vi "Set caseStructure Position and Size.vi"() -> ()   [LabVIEW 2012]
uses:
  <vilib>/Utility/miscctls.llb/LVBoundsTypeDef.ctl
panel:
  in  "Project Path":path
  in  "My Computer?":bool
  in  "Path":path
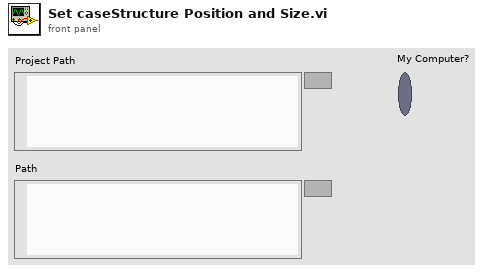
[diagram p1: front panel]
types:
  T1 = typedef "LVBoundsTypeDef.ctl" = cluster{"Width":u32, "Height":u32}
  T2 = typedef "LVPositionTypeDef.ctl" = cluster{"Left":i32, "Top":i32}
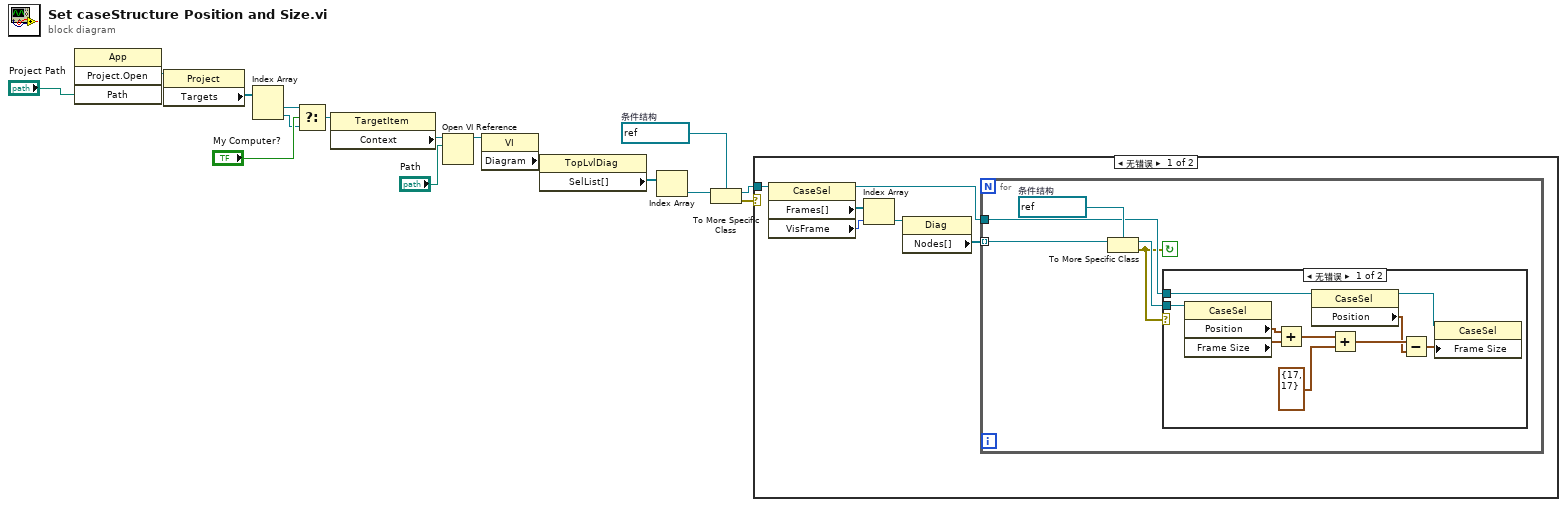
[diagram p0: block diagram]
diagram:
  w3 = refnum<vi> refnum  # 条件结构
  n1 = invoke class="App" method="Project.Open"("Path"="Project Path") -> ("Project:Open"=w15:refnum<vi>)  [unwired: 3 in, 3 out]
  n2 = property class="Project"(reference=w15) -> ("Targets"=w14:refnum<vi>[])  [unwired: 1 in, 2 out]
  n3 = Index Array(array=w14) -> (element #1=w11:refnum<vi>, element #2=w10:refnum<vi>)  [unwired: 2 in]
  n4 = Select(t=w11, s="My Computer?", f=w10) -> (s? t:f=w9:refnum<vi>)
  n5 = property class="TargetItem"(reference=w9) -> ("Context"=w8:refnum<vi>)  [unwired: 1 in, 2 out]
  n6 = Open VI Reference(application reference (local)=w8, vi path="Path") -> (vi reference=w7:refnum<vi>)  [unwired: 4 in, 1 out]
  n7 = property class="VI"(reference=w7) -> ("Diagram"=w6:refnum<vi>)  [unwired: 1 in, 2 out]
  n8 = property class="TopLvlDiag"(reference=w6) -> ("SelList[]"=w5:refnum<vi>[])  [unwired: 1 in, 2 out]
  n9 = Index Array(array=w5) -> (element=w4:refnum<vi>)  [unwired: 1 in]
  n10 = To More Specific Class(target class=w3, reference=w4) -> (specific class reference=w1:refnum<vi>, error out=w2:errorcluster)  [unwired: 1 in]
  n11 = case shown="无错误" w2 {
    tunnel: w1 -> [w22 _]
    frame No Error {
      n12 = property class="CaseSel"(reference=w22) -> (reference out=w19:refnum<vi>, "Frames[]"=w21:refnum<vi>[], "VisFrame"=w20:u32)  [unwired: 1 in, 1 out]
      n13 = Index Array(array=w21, index=w20) -> (element=w18:refnum<vi>)
      n14 = property class="Diag"(reference=w18) -> ("Nodes[]"=w17:refnum<vi>[])  [unwired: 1 in, 2 out]
      n15 = for {
        tunnel: w19 -> [w25]
        tunnel: w17 -> [w24] mode=indexing
        stop <- w23 continue-if-true
        w27 = refnum<vi> refnum  # 条件结构
        n16 = To More Specific Class(target class=w27, reference=w24) -> (specific class reference=w26:refnum<vi>, error out=w23:errorcluster)  [unwired: 1 in]
        n17 = case shown="无错误" w23 {
          tunnel: w26 -> [w37 _]
          tunnel: w25 -> [w31 _]
          frame No Error {
            n18 = property class="CaseSel"(reference=w37) -> ("Position"=w36:T2, "Frame Size"=w35:T1)  [unwired: 1 in, 2 out]
            n19 = Add(x=w36, y=w35) -> (x+y=w34:T1)
            n20 = property class="CaseSel"(reference=w31) -> (reference out=w30:refnum<vi>, "Position"=w28:T2)  [unwired: 1 in, 1 out]
            n21 = Add(x=w34, y=T1 {"Width"=17, "Height"=17}) -> (x+y=w32:T1)
            n22 = Subtract(x=w32, y=w28) -> (x-y=w29:T1)
            n23 = property class="CaseSel"(reference=w30, "Frame Size"=w29) -> ()  [unwired: 1 in, 2 out]
          }
          frame Error {
          }
        }
      }
    }
    frame Error {
    }
  }
